vi "motor direction on and off.vi"(8 "State 3":bool, 9 "State 2":bool, 10 "State 1":bool, 11 "State 0":bool) -> ()   [LabVIEW 2015]
panel:
  in  "FirstFound 3":bool=TRUE caption="FirstFound 8"
  out "Error Message 3":string
  out "error out 3":errorcluster
  in  "FirstFound 2":bool=TRUE caption="FirstFound 8"
  out "Error Message 2":string
  out "error out 2":errorcluster
  in  "FirstFound 1":bool=TRUE caption="FirstFound 8"
  out "Error Message 1":string
  out "error out 1":errorcluster
  in  "FirstFound 0":bool=TRUE caption="FirstFound 8"
  out "Error Message 0":string
  out "error out 0":errorcluster
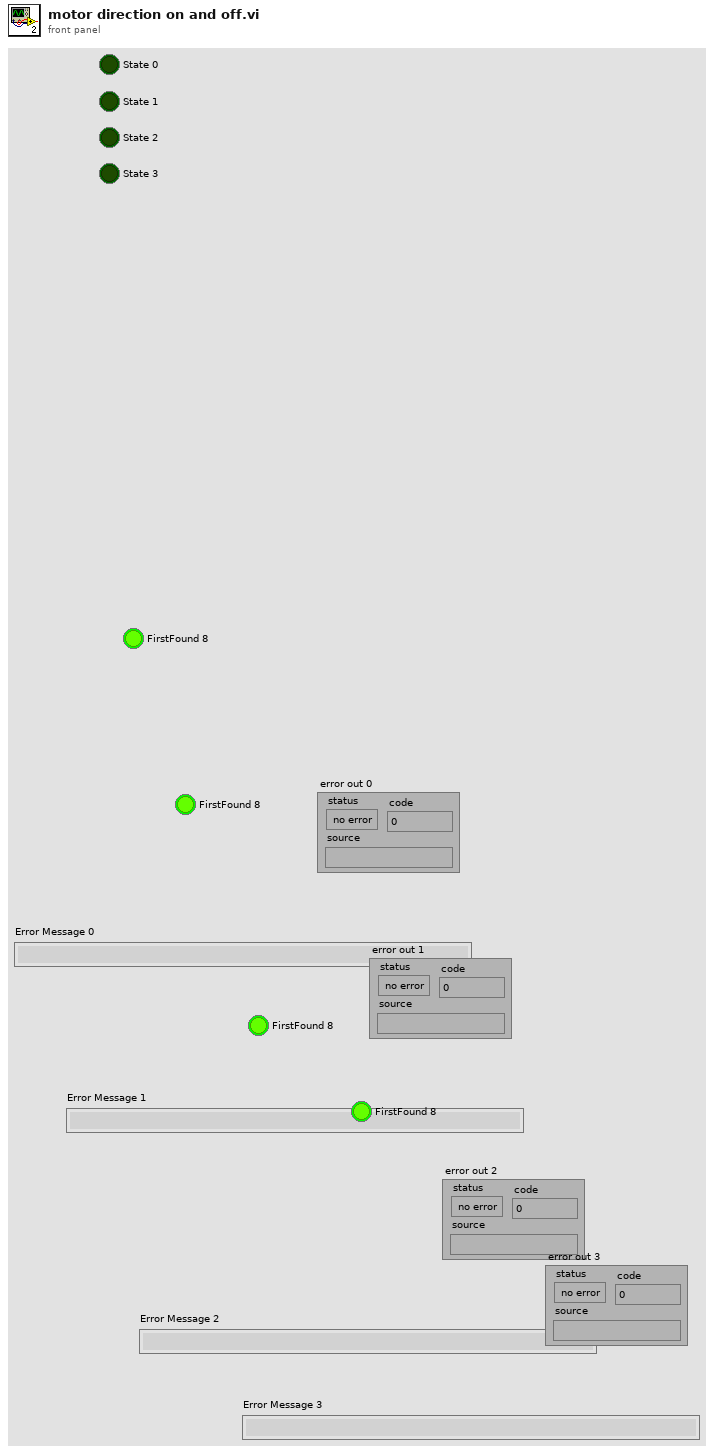
[diagram p1: front panel]
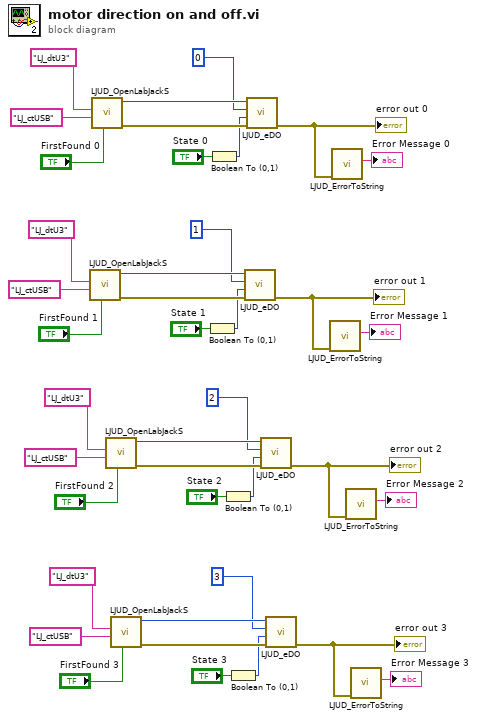
[diagram p0: block diagram]
diagram:
  n1 = call "LJUD_OpenLabJackS.vi"("FirstFound"="FirstFound 1", "ConnectionType"="LJ_ctUSB", "DeviceType"="LJ_dtU3") -> ("error out"=w25:errorcluster, "Handle"=w26:i32)  [unwired: 6 in, 1 out]
  n2 = call "LJUD_OpenLabJackS.vi"("FirstFound"="FirstFound 0", "ConnectionType"="LJ_ctUSB", "DeviceType"="LJ_dtU3") -> ("error out"=w35:errorcluster, "Handle"=w36:i32)  [unwired: 6 in, 1 out]
  n3 = call "LJUD_OpenLabJackS.vi"("FirstFound"="FirstFound 2", "ConnectionType"="LJ_ctUSB", "DeviceType"="LJ_dtU3") -> ("error out"=w15:errorcluster, "Handle"=w16:i32)  [unwired: 6 in, 1 out]
  n4 = call "LJUD_OpenLabJackS.vi"("FirstFound"="FirstFound 3", "ConnectionType"="LJ_ctUSB", "DeviceType"="LJ_dtU3") -> ("error out"=w5:errorcluster, "Handle"=w6:i32)  [unwired: 6 in, 1 out]
  n5 = Boolean To (0,1)(Boolean="State 1") -> (0, 1=w21:i16)
  n6 = Boolean To (0,1)(Boolean="State 0") -> (0, 1=w31:i16)
  n7 = Boolean To (0,1)(Boolean="State 2") -> (0, 1=w11:i16)
  n8 = Boolean To (0,1)(Boolean="State 3") -> (0, 1=w1:i16)
  n9 = call "LJUD_eDO.vi"("error in"=w25, "State"=w21, "Channel"=1 ("Channel 7"), "Handle In"=w26) -> ("error out"=w24:errorcluster)  [unwired: 6 in, 1 out]
  "error out 1" <- w24
  n10 = call "LJUD_eDO.vi"("error in"=w35, "State"=w31, "Channel"=0 ("Channel 7"), "Handle In"=w36) -> ("error out"=w34:errorcluster)  [unwired: 6 in, 1 out]
  "error out 0" <- w34
  n11 = call "LJUD_eDO.vi"("error in"=w15, "State"=w11, "Channel"=2 ("Channel 7"), "Handle In"=w16) -> ("error out"=w14:errorcluster)  [unwired: 6 in, 1 out]
  "error out 2" <- w14
  n12 = call "LJUD_eDO.vi"("error in"=w5, "State"=w1, "Channel"=3 ("Channel 7"), "Handle In"=w6) -> ("error out"=w4:errorcluster)  [unwired: 6 in, 1 out]
  "error out 3" <- w4
  n13 = call "LJUD_ErrorToString.vi"("error in"=w24) -> ("String"=→"Error Message 1":string)  [unwired: 10 in]
  n14 = call "LJUD_ErrorToString.vi"("error in"=w34) -> ("String"=→"Error Message 0":string)  [unwired: 10 in]
  n15 = call "LJUD_ErrorToString.vi"("error in"=w14) -> ("String"=→"Error Message 2":string)  [unwired: 10 in]
  n16 = call "LJUD_ErrorToString.vi"("error in"=w4) -> ("String"=→"Error Message 3":string)  [unwired: 10 in]
